vi "Get State Name.vi"(8 "error in (no error)":errorcluster, 11 "Waiting in":refnum<class "Waiting.lvclass">) -> (0 "error out":errorcluster, 2 "State Name":string, 3 "Waiting out":refnum<class "Waiting.lvclass">)   [LabVIEW 2013, in "Command Processor.lvlib" / "Waiting.lvclass"]
uses:
  Waiting.lvclass
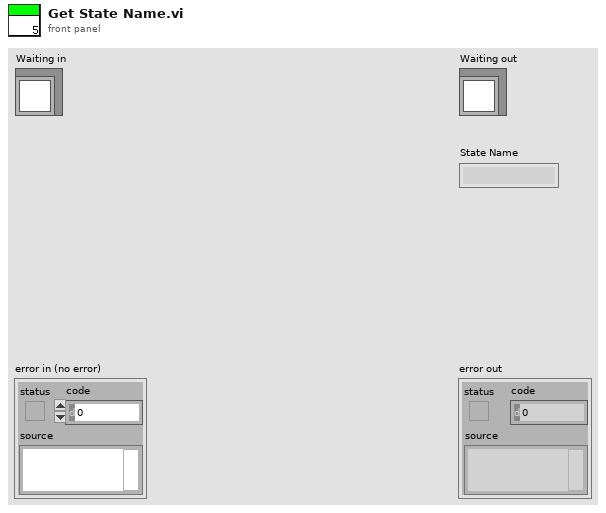
[diagram p1: front panel]
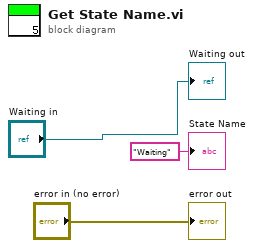
[diagram p0: block diagram]
diagram:
  "error out" <- "error in (no error)"
  "Waiting out" <- "Waiting in"
  "State Name" <- "Waiting" ("State Name")
